vi "TargetControllers.vi"() -> ()   [LabVIEW 2024]
uses:
  <vilib>/platform/TimedLoop/XDataNode/XDataNode.xnode
  <vilib>/Platform/TimedLoop/XDataNode/nitl_modes.ctl
  <vilib>/Platform/TimedLoop/XDataNode/XDNodeRunTimeDep.lvlib
  <vilib>/Platform/TimedLoop/XDataNode/wakeup.ctl
  <vilib>/Platform/TimedLoop/XDataNode/timing_clust.ctl
  <vilib>/Analysis/Matrix/NI_Matrix.lvlib
  subVIs_target/GlobalVariables.vi
  <vilib>/addons/Maxon Motor/EPOS2 CANopen/EPOS2 Support Files/Typedefs/EPOS2 Control Word PVM.ctl
  <vilib>/addons/Maxon Motor/EPOS2 CANopen/EPOS2 Library.lvlib
  <vilib>/Analysis/Matrix/Numeric/Conversions/Array To Matrix - RA2.vi
  <vilib>/addons/control/pid/NI_PID_pid.lvlib
  <vilib>/addons/control/pid/pid.llb/PID Output Rate Limiter (DBL Array).vi
  <vilib>/addons/Maxon Motor/EPOS2 CANopen/CANopen/sbCANopenBaseClass.lvclass
panel:
  out "Convert microsecond to second array":dbl[](array[numeric])
  out "Previous Tensions":dbl[](array[numeric])
  in  "Use pull-only friction compensation in feedforward control":bool=TRUE
  in  "Use linear tension/current model in feedforward control":bool=TRUE
  out "Motor velocities in ascending motor order":dbl[](array[numeric]) format="%.2f"
  out "Reinitialize PID all motors flags":bool[](array[boolean])
  out "maskForAllActiveMotors":bool[](array[boolean])
  out "NumTotalActiveMotors":i32
  out "Robot Control Mode Target Local":T1(radio)
  out "kneeActiveMotorNumbers":i32[](array[numeric])
  out "pelvisActiveMotorNumbers":i32[](array[numeric])
  out "trunkActiveMotorNumbers":i32[](array[numeric])
  out "NumActiveKneeMotors":i32
  out "NumActivePelvisMotors":i32
  out "NumActiveTrunkMotors":i32
  out "Velocity 5":dbl[](array[numeric])
  out "Velocity 3":dbl[](array[numeric])
  out "Velocity 2":dbl[](array[numeric])
  out "Motor order":i32[](array[numeric])=[3, 6, 9, 12, 2, 7, 8, 13, 4, 5, 10, 11, 1, 14]
  out "maskForKneeMotors":bool[](array[boolean])
  out "maskForPelvisMotors":bool[](array[boolean])
  out "maskForTrunkMotors":bool[](array[boolean])
  out "Vicon Sync":dbl format="%0.2f"
  out "True_Knees":bool=TRUE
  out "final current":dbl[](array[numeric])
  out "Pelvis Forces Enabled":bool=TRUE
  out "canERROR":errorcluster[](array[cluster])
  in  "CANcurrent 2":dbl[](array[numeric])
  out "Low-Level Controller Finished Late?":bool
  out "CANcurrent":dbl[](array[numeric])
  out "Read Late":bool
  out "Read Time":i64
  out "I32":i32
  out "Write Late":bool
  out "Write Time":i64
  out "canID":refnum<class "sbCANopenBaseClass.lvclass">[](array[class])
  out "nMotorsCAN":i32
  out "AcT":dbl[](array[numeric])
  out "Period_HL":dbl format="%.2f"
  out "Current Tension":dbl[](array[numeric])
  in  "Stop":bool
  out "UseATI":bool
  out "PID loop duration [us]":i64
  # "Note before running this VI:\n1. Ensure correct motors are selected \nusing MotorsToUse.\n2. Connected load cells should have \nthe same order as MotorsToUse.\n\n-------- Do appropriate transformation in CONSTS LL and HL VIs -----------\n(especially MotorsPos_wrt_Markers )"
  # "Motor Order \n(Trunk, Pelvis, Pelvis_M, Leg)\n3\n6\n9\n12\n2\n7\n8\n13\n4\n5\n10\n11\n1\n14"
  # "This part reads\nmotors in order from\nTrunk, pel, etc, and not\nthe motor # order 1-14. \n\nAlso, the code motor number\nis 1 less than the labeled motor \nnumber (e.g., motor 1 is 0)."
types:
  T1 = enum32{"Idle", "Constant", "Live Forces", "Single Motor", "Constant Feedforward"}
  T2 = typedef "EPOS2 Library.lvlib/EPOS2 Control Word PVM.ctl" = cluster{"Switch On":bool, "Enable Voltage":bool, "Quick Stop":bool, "Enable Operation":bool, "Reserved 0":bool, "Reserved 1":bool, "Reserved 2":bool, "Fault Reset":bool, "Halt":bool}
  T3 = typedef "XDNodeRunTimeDep.lvlib/timing_clust.ctl" = cluster{"Expected End [f-1]":u64, "Actual End [f-1]":u64, "Finished Late? [f-1]":bool, "Expected End [i-1]":u64, "Actual End [i-1]":u64, "Finished Late? [i-1]":bool, "Expected Start [i]":u64, "Actual Start [i]":u64, "Expected Start [f]":u64, "Actual Start [f]":u64, "Source Name":string, "Structure Name":string, "Period":i64, "Deadline":i64, "Offset":i64, "Start":i64, "Priority":i32, "Timeout":i32, "Mode":T4, "Wakeup Reason":T5, "Error":errorcluster, "Source Type":string, "Secondary Source Type":string, "Global End Time":u64, "Global Start Time":u64, "Frame Duration":u64, "Iteration Duration":u64, "Assigned CPU":i32, "I/O Scan Engine Mode":u32}
  T4 = typedef "XDNodeRunTimeDep.lvlib/nitl_modes.ctl" = enum32{"No Change", "Process missed periods, maintain original phase", "Discard missed periods, maintain original phase", "Process missed periods, ignore original phase", "Discard missed periods, ignore original phase"}
  T5 = typedef "XDNodeRunTimeDep.lvlib/wakeup.ctl" = enum32{"Normal", "Aborted", "Asynchronous wakeup", "Timing source error", "Timed loop error", "Timeout"}
  T6 = typedef "constants_LL.ctl" = cluster{"zero array":dbl[], "decRate_ff":dbl[], "Motor constants":dbl[], "PID gains":cluster{"proportional gain (Kc)":dbl, "integral time (Ti, min)":dbl, "derivative time (Td, min)":dbl}[], "decRate _fb":dbl[], "PID_OP_upLim":dbl, "nMotors":i32, "PID_betas":dbl[], "filtOrder":i32, "filtLowCutFreq":dbl, "filtSamplFreq":dbl, "whichMotors":i32[], "nMotors 1":i32, "nMotors 2":i32, "Motor constants pel":dbl[], "Motor constants trunk":dbl[], "whichMotors 1":i32[], "whichMotors 2":i32[], "zero array pel":dbl[], "decRate_ff pel":dbl[], "decRate _fb pel":dbl[], "PID_betas pel":dbl[], "whichMotors 3":i32[], "nMotors 3":i32, "Motor constants knees":dbl[], "zero array knees":dbl[], "decRate_ff knees":dbl[], "decRate _fb knees":dbl[], "PID_betas knees":dbl[]}
  T7 = typedef "NI_Matrix.lvlib/RealMatrix.ctl" = dbl[][]
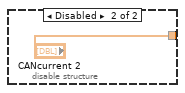
[diagram p2: hidden frame]
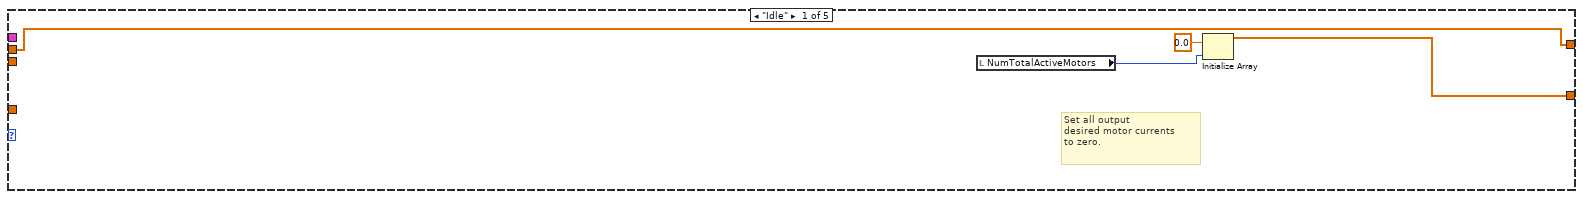
[diagram p4: hidden frame]
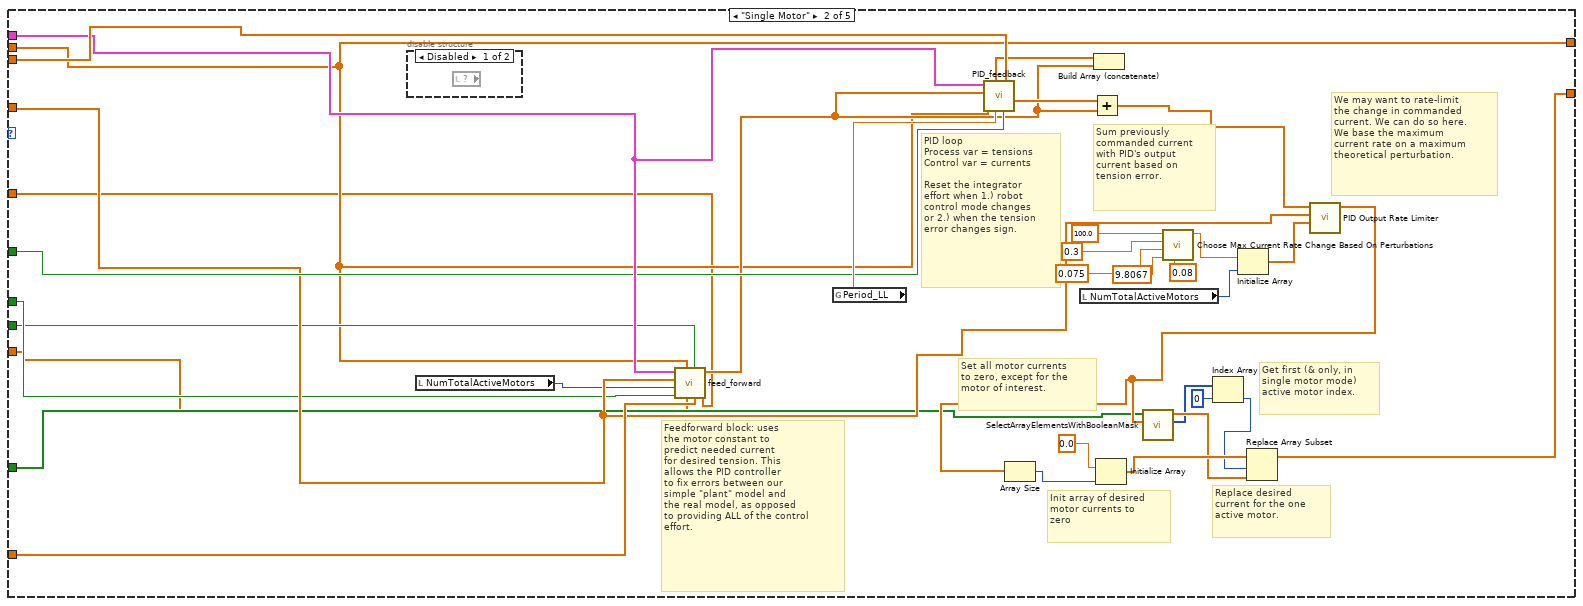
[diagram p5: hidden frame]
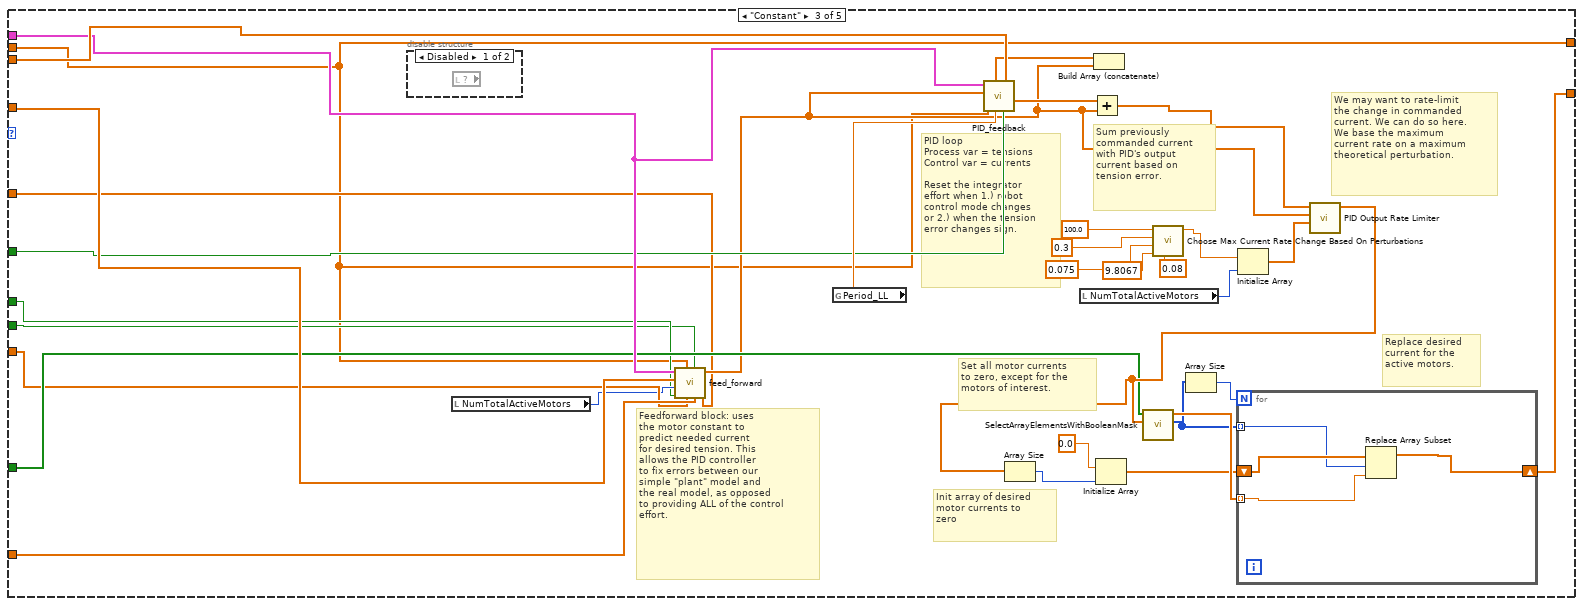
[diagram p7: hidden frame]
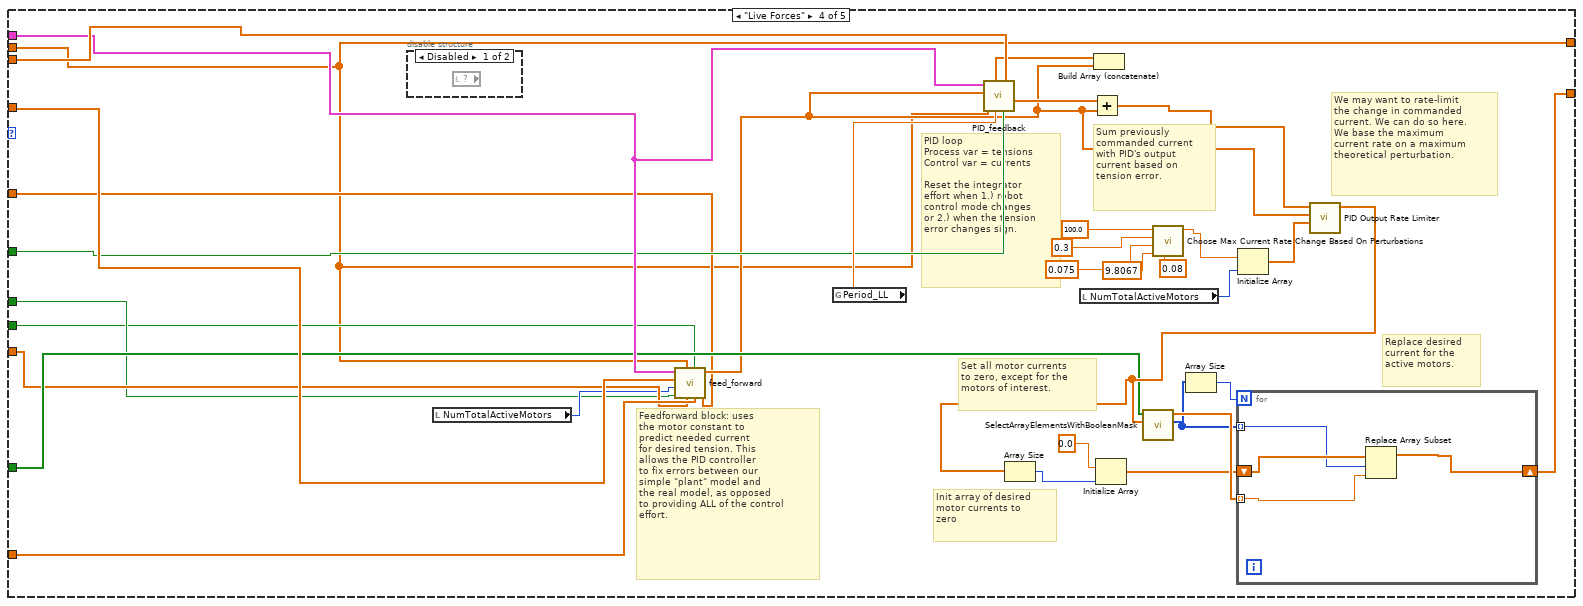
[diagram p9: hidden frame]
diagram:
  n1 = flat-sequence {
    tunnel: [w64] -> w17
    tunnel: [w62] -> w16
    tunnel: [w58] -> w15
    tunnel: [w56] -> w14
    tunnel: [w55] -> w13
    tunnel: [w49] -> w10
    tunnel: [w48] -> w9
    tunnel: w17 -> [w113]
    tunnel: w16 -> [_]
    tunnel: w15 -> [_]
    tunnel: w14 -> [w87]
    tunnel: w13 -> [w86]
    tunnel: [w87] -> w12
    tunnel: [w86] -> w11
    tunnel: w10 -> [w85]
    tunnel: w9 -> [w96]
    tunnel: [w97] -> w8
    tunnel: [w85] -> w7
    tunnel: [w96] -> w6
    tunnel: [w92] -> w2
    tunnel: [w91] -> w1
    tunnel: w12 -> [w383]
    tunnel: w11 -> [w382]
    tunnel: w8 -> [w379]
    tunnel: w7 -> [w378]
    tunnel: w6 -> [w377]
    tunnel: [w379] -> w5
    tunnel: [w376] -> w4
    tunnel: [w375] -> w3
    tunnel: w2 -> [w374]
    tunnel: w1 -> [w373]
    tunnel: w5 -> [w394]
    tunnel: w4 -> [w393]
    tunnel: w3 -> [w392]
    frame #0 {
      w44 = TRUE
      w46 = TRUE
      w57 = refnum<k21> "LEDTrust"  # DAQmx Task Name
      w63 = dbl[][] [[-1.3915001098602042, -96.36354731251453, 1.4901268489488144, 95.80055650167623, 0.11513435812043361, -0.20957134618573833], [-0.15155726034970227, -54.43374806490713, -0.3124157679711426, -56.28095342773552, -2.859114029977124, 103.37942505940691], [135.67639082873404, -1.227548634927782, 136.40217860533392, -2.4579984396752574, 136.3751481938431, -5.182267660606754], [-2.217796179322478, -0.3587679442089546, 2.274983310429265, -0.42200713926637096, -0.04878150351528989, 0.7012551466653533], [-1.289313295754956, 0.6617253849307168, -1.3327588652039173, -0.632747230304039, 2.4993576210336226, -0.09390740213198005], [-0.003620332273444647, -1.4342719694352277, -0.021014064916045613, -1.406174049990865, 0.009761043049281059, -1.3430405096008415]]  # Callibration Matrix Sensor ID: FT5769
      w61 = FALSE ("ATIConnected")
      # "This is the startup frame. \nAll code in this frame runs once \nat startup."
      # "At startup, we reinitialize\nthe PID controller to zero\nout the integrator."
      # "The current CAN Initialize assumes \na fixed order of motors, e.g. the first 4 are\n for the trunk, the next 8 are for the \npelvis, and the last two are for the knees. \nI added an int[] output that reports the order\nof the motor numbers."
      # "The low-level (LL) constants include \nmotor constants, PID constants for the tension loop\n, other?"
      # "CAN_motorselect.vi selects only\nthe motors we need given the flags \nof UsingTrunk, UsingPelvisPlanar, \nUsingPelvisMoments, and UsingKnees.\nOne idea: turn them all on and only \nwrite non-zero currents to those we need."
      # "Can_Initialize3.vi appears to\ninitialize all 14 motors"
      # "Low Level Constants: \nPID parameters\nMotor constants"
      # "LED Trust"
      # "Operation Mode\nEnabled"
      # "Legs"
      # "Pelvis-Forces/Moments"
      # "Pelvis-Planar"
      # "Trunk"
      # "Operation Mode\nDisabled"
      # "Initialize/\nPreOperation"
      n2 = call "CAN_initialize3.vi"() -> ("Array 2"=w41:errorcluster[], "Array"=w43:refnum<class "sbCANopenBaseClass.lvclass">[], "Motor order"=→"Motor order":i32[])  [unwired: 3 in]
      n3 = shared-variable "NI-PXIe8880-2F170198\\variables_AlwaysInUse - networkPublished.lvlib\\Use Vicon"(w61) -> ()  [unwired: 1 in, 1 out]
      n4 = shared-variable "NI-PXIe8880-2F170198\\variables_ToSetPID - networkPublished.lvlib\\SetPID"(w61) -> ()  [unwired: 1 in, 1 out]
      n5 = shared-variable "NI-PXIe8880-2F170198\\variables_AlwaysInUse - networkPublished.lvlib\\Use ATI"(w61) -> ()  [unwired: 1 in, 1 out]
      n6 = call "CAN_MotorSelect.vi"("Trunk"=TRUE, "Nodes In"=w43, "Pelvis"=w46, "Pelvis_Moments"=TRUE, "Legs"=w44, "Error In"=w41) -> ("maskForTrunkMotors"=w25:bool[], "Nodes Out"=w42:refnum<class "sbCANopenBaseClass.lvclass">[], "nMotorsCAN"=w39:i32, "maskForKneeMotors"=w23:bool[], "CANmotorsuse"=w38:bool[], "Error Out"=w40:errorcluster[], "maskForPelvisMotors"=w24:bool[])  [unwired: 3 in]
      "nMotorsCAN" <- w39
      "maskForTrunkMotors" <- w25
      "maskForPelvisMotors" <- w24
      "maskForKneeMotors" <- w23
      n7 = local read "Motor order"() -> (w33:i32[])
      n8 = for {
        N: w39 -> [_]
        tunnel: [w79] -> w53 mode=indexing
        tunnel: w42 -> [w78] mode=indexing
        tunnel: w40 -> [w77] mode=indexing
        tunnel: [w75] -> w54 mode=indexing
        n9 = Wait (ms)(milliseconds to wait=u32 100) -> ()  [unwired: 1 out]
        n10 = call "CAN_enableOFF.vi"("error in (no error)"=w77, "Current"=0, "sbCANopenBaseClass in"=w78) -> ("error out"=w79:errorcluster, "CANopen Session Out"=w75:refnum<class "sbCANopenBaseClass.lvclass">)  [unwired: 1 in]
      }
      n11 = local write "Stop"(FALSE ("Stop")) -> ()
      n12 = call "SelectArrayElementsWithBooleanMask.vi"("InputArray"=w33, "BooleanMaskArray"=w24) -> ("OutputArray"=→"pelvisActiveMotorNumbers":dbl[])  [unwired: 8 in, 1 out]
      n13 = call "SelectArrayElementsWithBooleanMask.vi"("InputArray"=w33, "BooleanMaskArray"=w25) -> ("OutputArray"=→"trunkActiveMotorNumbers":dbl[])  [unwired: 8 in, 1 out]
      n14 = call "SelectArrayElementsWithBooleanMask.vi"("InputArray"=w33, "BooleanMaskArray"=w23) -> ("OutputArray"=→"kneeActiveMotorNumbers":dbl[])  [unwired: 8 in, 1 out]
      n15 = shared-variable "NI-PXIe8880-2F170198\\variables_AlwaysInUse - networkPublished.lvlib\\directTension"(0.0 ("directTension")) -> ()  [unwired: 1 in, 1 out]
      n16 = call "Sum_True_Elements_In_Boolean_Array.vi"("InputBooleanArray"=w23) -> ("NumTruesInArray"=w27:i32)  [unwired: 10 in]
      "NumActiveKneeMotors" <- w27
      n17 = call "Sum_True_Elements_In_Boolean_Array.vi"("InputBooleanArray"=w25) -> ("NumTruesInArray"=w29:i32)  [unwired: 10 in]
      "NumActiveTrunkMotors" <- w29
      n18 = call "Sum_True_Elements_In_Boolean_Array.vi"("InputBooleanArray"=w24) -> ("NumTruesInArray"=w28:i32)  [unwired: 10 in]
      "NumActivePelvisMotors" <- w28
      n19 = Bundle By Name(cluster=T2 {"Switch On"=TRUE, "Enable Voltage"=TRUE, "Quick Stop"=TRUE, "Enable Operation"=TRUE, "Reserved 0"=FALSE, "Reserved 1"=FALSE, "Reserved 2"=FALSE, "Fault Reset"=FALSE, "Halt"=FALSE} ("Control Word"), "Switch On"=TRUE) -> (w50:T2)
      n20 = Add(x=w29, y=w28) -> (x+y=w26:i32)
      n21 = for {
        N: w39 -> [_]
        tunnel: w54 -> [w70]
        tunnel: w53 -> [w69]
        tunnel: w50 -> [w65]
        tunnel: [w67] -> w49 mode=indexing
        tunnel: [w66] -> w48 mode=indexing
        i -> [w71]
        # "Writes current = 0 to all motors.\nTURNING ON the first 4 boolean values \nin the \"otuput cluster\" variable of CAN_MotorControl2.vi\nputs the CAN node in the correct mode for reading\nPDOs (current, velocity, position, etc.)"
        n22 = Wait (ms)(milliseconds to wait=u32 100) -> ()  [unwired: 1 out]
        n23 = Index Array(array=w70, index=w71) -> (element=w74:refnum<class "sbCANopenBaseClass.lvclass">)
        n24 = Index Array(array=w69, index=w71) -> (element=w68:errorcluster)
        n25 = call "CAN_MotorControl2.vi"("output cluster"=w65, "sbCANopenBaseClass in"=w74, "Current"=0, "error in (no error)"=w68) -> ("CANopen Session Out"=w67:refnum<class "sbCANopenBaseClass.lvclass">, "error out"=w66:errorcluster)  [unwired: 2 in]
      }
      n26 = Add(x=w26, y=w27) -> (x+y=w18:i32)
      "NumTotalActiveMotors" <- w18
      n27 = Or(x=w25, y=w24) -> (x .or. y?=w22:bool[])
      n28 = Or(x=w22, y=w23) -> (x .or. y?=→"maskForAllActiveMotors":bool[])
      n29 = local read "NumActiveKneeMotors"() -> (w34:i32)
      n30 = local read "NumActivePelvisMotors"() -> (w35:i32)
      n31 = local read "NumActiveTrunkMotors"() -> (w36:i32)
      n32 = Initialize Array(TRUE, w18) -> (→"Reinitialize PID all motors flags":bool[])
      n33 = call "constants_LL.vi"("NumKneeMotorsInUse"=w34, "NumPelvisMotorsInUse"=w35, "MotorsInUse"=w38, "NumTrunkMotorsInUse"=w36) -> ("Constants LL"=w64:T6)  [unwired: 7 in]
      n34 = call-poly <vilib>:"Array To Matrix.vi"("Real 2D Array"=w63) -> ("Real Matrix"=w62:T7)
      n35 = call <vilib>:"DAQmx Start Task.vi"("task/channels in"=w57) -> ("task out"=w56:refnum<k21>, "error out"=w55:errorcluster)  [unwired: 13 in]
      n36 = Tick Count (ms)() -> (millisecond timer value=w58:u32)
      "Pelvis Forces Enabled" <- w46
      "True_Knees" <- w44
    }
    frame #1 {
      w93 = i64 5000  # @ 200Hz
      w110 = i64 2500  # @ 1000Hz
      # "Used to convert N/us to N/s"
      # "Period for reading \nCAN data (in us)"
      # "This is the primary frame of the code. \nAll timed loops are in this frame. \nFrom top to bottom:\n1.) Write CAN loop: sends desired motor currents to the motor controllers.\n2.) Read CAN loop: seems to only read motor velocity (RPM). Note that tension sensors \nare read in the LL controller loop. \n3.)  Low level controller loop: based on desired tensions, uses feedforward control \n(special motor constant * current = tension) and PID feedback control on tensions to set desired motor\ncurrents."
      # "All motor currents are \ninitialized at 0 A"
      # "Here is the output of CAN nodes \nwith all the motors. All of these motors\nare in Current mode and are enabled."
      # "Rob 3/7/23: Was 2000 us delay (500Hz), \nslowing to 2,500 us delay (400 Hz)"
      # "Rob 3/7/23: Was 5000 us delay, \nslowing to 10,000."
      # "Global Variables are made by saving a separate VI\nright-click and explore to see it"
      # "These are typedefs below.\nAdjustable in project list"
      # "d1: time, cT, dT\n\nd4: d1, fN, data, QP_error\n\ndata: dFM, cFM, dFMNF, ..."
      # "About 750Hz"
      # "CAN protocol does not like local variables for some reason. Use these long wires to connect"
      # "uses 0 to 13 for motors"
      # "sec"
      n37 = node-c288(i64 1000 ("Period")) -> (w95:T3)  [unwired: 3 in]
      n38 = timed-loop {
        timing: w95 -> [_]
        timing-out: [_] -> w94
        tunnel: w85 -> [w122]
        tunnel: w96 -> [w123]
        stop <- w130 stop-if-true
        # "The motor velocities are in the order of the NodeIDs. \nRe-order to ascending motor numbers."
        # "GearRatio"
        # "Read CAN"
        n39 = node-c288() -> (→"Read Late":bool, →"Read Time":i64)  [unwired: 1 in, 1 out]
        n40 = local read "NumTotalActiveMotors"() -> (w124:i32)
        n41 = for {
          N: w124 -> [_]
          tunnel: [w140] -> w126 mode=indexing
          tunnel: w122 -> [w139] mode=indexing
          tunnel: w123 -> [w138] mode=indexing
          n42 = call-dynamic "sdCANopenPDOread.vi"("error in (no error)"=w138, "PDO Number"=u8 1, "sbCANopenBaseClass in"=w139) -> ("Data"=w141:u8[])  [unwired: 6 in, 2 out]
          n43 = Split 1D Array(array=w141, index=4) -> (first subarray=w137:u8[])  [unwired: 1 out]
          n44 = call <vilib>:"sdCANutility4xU8toI32.vi"("Array 4 U8"=w137) -> ("I32"=w140:i32)
          "I32" <- w140
        }
        n45 = Initialize Array(14.0 ("element"), w124) -> (w127:dbl[])
        n46 = local read "NumTotalActiveMotors"() -> (w119:i32)
        n47 = local read "Motor order"() -> (w120:i32[])
        n48 = Divide(x=w126, y=w127) -> (x/y=w121:dbl[])
        n49 = Initialize Array(0.0 ("element"), w119) -> (w117:dbl[])
        n50 = for {
          tunnel: w121 -> [w132] mode=indexing
          tunnel: w120 -> [w136] mode=indexing
          shift-right: [w131] -> w116
          shift-left: w117 -> [w134]
          # "When storing in ascending motor\norder, the index is just the motor \nnumber - 1."
          n51 = Subtract(x=w136, y=1) -> (x-y=w133:i32)
          n52 = Replace Array Subset(array=w134, new element=w132, index=w133) -> (w131:dbl[])
        }
        "Motor velocities in ascending motor order" <- w116
        n53 = local read "Stop"() -> (w130:bool)
        n54 = node-c288() -> ()  [unwired: 1 in, 1 out]
      }
      n55 = node-c288() -> (w105:T3)  [unwired: 3 in]
      n56 = Bundle By Name(cluster=T2 {"Switch On"=TRUE, "Enable Voltage"=TRUE, "Quick Stop"=TRUE, "Enable Operation"=TRUE, "Reserved 0"=FALSE, "Reserved 1"=FALSE, "Reserved 2"=FALSE, "Fault Reset"=FALSE, "Halt"=FALSE} ("Control Word"), "Switch On"=TRUE) -> (w101:T2)
      n57 = timed-loop {
        tunnel: w96 -> [w159]
        tunnel: [w157] -> _
        timing: w105 -> [_]
        timing-out: [_] -> w104
        tunnel: w101 -> [w155]
        tunnel: w85 -> [w160]
        tunnel: [w156] -> _
        stop <- w154 stop-if-true
        # "Here, the latest computed motor currents are \nsent to each motor via the CAN communication protocol."
        # "Write CAN"
        n58 = node-c288() -> (→"Write Late":bool, →"Write Time":i64)  [unwired: 1 in, 2 out]
        n59 = disable-structure shown="Enabled" {
          disable-tunnel: [w162 "CANcurrent 2"] -> w152
          frame Enabled {
            n60 = local read "CANcurrent"() -> (w162:dbl[])
          }
          frame Disabled {
          }
        }
        n61 = local read "nMotorsCAN"() -> (w153:i32)
        n62 = for {
          N: w153 -> [_]
          tunnel: [w170] -> w156 mode=indexing
          tunnel: [w171] -> w157 mode=indexing
          tunnel: w160 -> [w172] mode=indexing
          tunnel: w159 -> [w173] mode=indexing
          tunnel: w155 -> [w169]
          tunnel: w152 -> [w168] mode=indexing
          n63 = call "CAN_MotorControl2.vi"("output cluster"=w169, "sbCANopenBaseClass in"=w172, "Current"=w168, "error in (no error)"=w173) -> ("CANopen Session Out"=w170:refnum<class "sbCANopenBaseClass.lvclass">, "error out"=w171:errorcluster)  [unwired: 2 in]
        }
        "canID" <- w156
        "canERROR" <- w157
        n64 = local read "Stop"() -> (w154:bool)
        n65 = node-c288() -> ()  [unwired: 1 in, 1 out]
      }
      n66 = local read "NumTotalActiveMotors"() -> (w83:i32)
      n67 = local read "NumTotalActiveMotors"() -> (w89:i32)
      n68 = Initialize Array(1000000.0 ("element"), w83) -> (→"Convert microsecond to second array":dbl[])
      n69 = call <vilib>:"DAQmx Start Task.vi"("task/channels in"=refnum<k21> "SCI_TenSen") -> ("task out"=w100:refnum<k21>, "error out"=w99:errorcluster)  [unwired: 13 in]
      n70 = Initialize Array(0.0 ("element"), w89) -> (w88:dbl[])
      n71 = node-c288(w110) -> (w115:T3)  [unwired: 3 in]
      n72 = timed-loop "Timed Loop" {
        timing: w115 -> [_]
        timing-out: [_] -> w114
        shift-right: [w194] -> _
        shift-left: w88 -> [w207]
        shift-right: [w203] -> _
        shift-left: w113 -> [w212]
        tunnel: w99 -> [w188]
        tunnel: [w206] -> w91
        shift-right: [w205] -> w92
        shift-left: w100 -> [w205]
        stop <- "Stop" stop-if-true
        # "Do a \"quick and dirty\" approximation of \nchange in desired tension, in units of \nN/second. We approximate the loop time \nwith the previous loop time."
        # "Desired tensions [N]"
        # "Only read velocities IF we're using the pull comp. \nOtherwise, output 0 velocities.\nPROBLEM: reading is VERY slow, so if we activate this, \nour control loop performance tanks. Need to switch to PDO reads, currently SDO."
        # "CANcurrent: the \nvalues sent to the\nmotors over CAN."
        # "Our CAN nodes are \nordered in a certain way, \nwhereas our desired currents\nare ordered in ascending\norder. We must reorder them to\nmatch the CAN node order."
        # "Set the current robot control mode state.\n\nAlso, determine whether or not the robot high-level \ncontroller has switched states. We will use this information\nas whenever we change states, we want to zero the \nPID integrator effort. If the state has changed, output\n\"true\" to indicate that we want to reset the integrator."
        # "The ActiveMotorsFlags is a boolean mask\nwith dimension 14x1. All motors with a \nfalse will have their desired currents set to\n0. Note that this flag is set in the HostMain\nVI on the PC and depends on the robot \ncontrol mode."
        # "This is a \"friction compensation\"\nTENSION that was never fully \nimplemented."
        # "Below: motor selection masks\nfor all of the different robot modes."
        # "Convert from the int version of \nthe robot control mode (a global variable)\nback to a radio button format for clarity."
        # "DesiredTensionsX, where X is Trunk, \nPelvis, or Knees is a double array \nwith the number of elements equal to \nthe number of needed motors for that \nsegment. The"
        # "Feedforward motor\nfriction compensation \nin V (set to 0)"
        # "Here, tension\nvector is ordered\nby strain gauge \nnumber: 1,2,3,4,...\nand is thus \nin ascending\norder."
        # "This case structure determines desired currents for ALL motors. All motors \nnot included in the relevant state's motor mask will receive desired currents \nof zero."
        # "The DAQ is running\nthe \"SCI_TenSen\" \n(tension sensing) \ntask, meaning it \nwill read the tension\nsensors. The task \nname is set above (trace the Refnum in\ninput to \nAnalog_IP_Data.vi)"
        # "fix this"
        # "Current tension is initially read here!"
        # "Please be aware that ATI not considered for UseATI=true"
        # "Low Level Tension Controller"
        n73 = node-c288() -> (→"PID loop duration [us]":i64, →"Low-Level Controller Finished Late?":bool)  [unwired: 1 in]
        n74 = shared-variable "NI-PXIe8880-2F170198\\variables_AlwaysInUse - networkPublished.lvlib\\Use ATI"() -> (→"UseATI":bool)  [unwired: 1 in, 1 out]
        n75 = shared-variable "NI-PXIe8880-2F170198\\variables_ToSetPID - networkPublished.lvlib\\SetPID"() -> (w211:bool)  [unwired: 1 in, 1 out]
        n76 = case shown="True" w211 {
          tunnel: w212 -> [w222 w225]
          tunnel: [w222 w224] -> w203
          frame False {
          }
          frame True {
            n77 = shared-variable "NI-PXIe8880-2F170198\\variables_ToSetPID - networkPublished.lvlib\\pidGains"() -> (w223:dbl[])  [unwired: 1 in, 1 out]
            n78 = call "SetPIDGains.vi"("pidGains"=w223, "Constants LL in"=w225) -> ("Constants LL out"=w224:T6)  [unwired: 9 in]
          }
        }
        n79 = local read "Robot Control Mode Target Local"() -> (w197:T1)
        n80 = shared-variable "NI-PXIe8880-2F170198\\variables_Unity_Data.lvlib\\RobotControlModeAsInt"() -> (w198:i32)  [unwired: 1 in, 1 out]
        "Robot Control Mode Target Local" <- w198
        n81 = Not Equal?(x=w198, y=w197) -> (x != y?=w196:bool)
        n82 = call "Analog_IP_Data.vi"("Refnum in"=w205, "error in (no error)"=w188, "Constants LL"=w203) -> ("Tension Sensors Data"=w195:dbl[], "error out"=w206:errorcluster, "Vicon Sync"=→"Vicon Sync":dbl)  [unwired: 1 in, 5 out]
        "Current Tension" <- w195
        "AcT" <- w195
        n83 = local read "Motor velocities in ascending motor order"() -> (w185:dbl[])
        n84 = shared-variable "NI-PXIe8880-2F170198\\variables_Unity_Data.lvlib\\DesiredTensionsInAscendingMotorOrder"() -> (w182:dbl[])  [unwired: 1 in, 1 out]
        n85 = local read "Previous Tensions"() -> (w181:dbl[])
        n86 = shared-variable "NI-PXIe8880-2F170198\\variables_Unity_Data.lvlib\\AllCurrentTensions"(w195) -> ()  [unwired: 1 in, 1 out]
        n87 = local read "Convert microsecond to second array"() -> (w177:dbl[])
        n88 = local read "PID loop duration [us]"() -> (w180:i64)
        n89 = Subtract(x=w182, y=w181) -> (x-y=w179:dbl[])
        n90 = local read "Robot Control Mode Target Local"() -> (w202:T1)
        n91 = local read "NumTotalActiveMotors"() -> (w201:i32)
        n92 = shared-variable "NI-PXIe8880-2F170198\\variables_Unity_Data.lvlib\\ActiveMotorsFlags"() -> (w199:bool[])  [unwired: 1 in, 1 out]
        n93 = Divide(x=w179, y=w180) -> (x/y=w178:dbl[])
        n94 = Multiply(x=w178, y=w177) -> (x*y=w176:dbl[])
        n95 = Initialize Array(40.0 ("element"), w201) -> (w200:dbl[])
        n96 = case shown="\"Constant Feedforward\"" w202 {
          tunnel: [w227 w262 w278 w314 w349] -> w194
          tunnel: w207 -> [_ w243 w294 w330 w360]
          tunnel: w195 -> [_ w261 w293 w329 _]
          tunnel: w203 -> [_ w259 w291 w327 w358]
          tunnel: w182 -> [w226 w231 w263 w299 w335]
          tunnel: w200 -> [_ w260 w292 w328 w359]
          tunnel: w199 -> [_ w242 w281 w317 w352]
          tunnel: w196 -> [_ w244 w282 w318 _]
          tunnel: w185 -> [_ w233 w268 w304 w339]
          tunnel: "Use linear tension/current model in feedforward control" -> [_ w234 w266 w302 _]
          tunnel: "Use pull-only friction compensation in feedforward control" -> [_ w232 w265 w301 _]
          tunnel: [w226 w231 w263 w299 w335] -> w183
          tunnel: w176 -> [_ w230 w264 w300 w336]
          frame "Idle" {
            # "Set all output \ndesired motor currents\nto zero."
            n97 = local read "NumTotalActiveMotors"() -> (w228:i32)
            n98 = Initialize Array(0.0 ("element"), w228) -> (w227:dbl[])
          }
          frame "Single Motor" {
            # "Replace desired\ncurrent for the one \nactive motor."
            # "Init array of desired \nmotor currents to \nzero"
            # "Get first (& only, in\nsingle motor mode)\nactive motor index."
            # "We may want to rate-limit\nthe change in commanded \ncurrent. We can do so here.\nWe base the maximum \ncurrent rate on a maximum\ntheoretical perturbation."
            # "Sum previously \ncommanded current\nwith PID's output \ncurrent based on \ntension error."
            # "PID loop\nProcess var = tensions\nControl var = currents\n\nReset the integrator\neffort when 1.) robot\ncontrol mode changes \nor 2.) when the tension\nerror changes sign."
            # "Feedforward block: uses\nthe motor constant to \npredict needed current \nfor desired tension. This\nallows the PID controller\nto fix errors between our \nsimple \"plant\" model and \nthe real model, as opposed\nto providing ALL of the control\neffort."
            # "Set all motor currents\nto zero, except for the \nmotor of interest."
            n99 = disable-structure shown="Disabled" {
              frame Disabled {
                n100 = local read item#-1() -> ()  [unwired: 1 out]
              }
              frame Enabled {
              }
            }
            n101 = local read "NumTotalActiveMotors"() -> (w235:i32)
            n102 = call "feed_forward.vi"("Desired tension velocities [N/s]"=w230, "frictionCompensationTensions"=w260, "Use pull-only friction compensation in feedforward"=w232, "Motor velocities (rpm)"=w233, "DesiredTensionsInAscendingMotorOrder"=w231, "Use linear tension/current modle in feedforward"=w234, "Num Total Active Motors"=w235, "lastCommandedMotorCurrent"=w243, "Constants LL"=w259) -> ("feedforwardPredictedMotorCurrents"=w241:dbl[])  [unwired: 2 in]
            n103 = global read "GlobalVariables.vi" "Period_LL"() -> (w257:dbl)
            n104 = call "PID_feedback.vi"("Reset PID and integrator Flag"=w244, "currentTensions"=w261, "dt (s)"=w257, "desiredTensions"=w231, "feedforwardCurrentsIn"=w241, "Constants LL"=w259) -> ("pidCurrentsOut"=w258:dbl[])  [unwired: 5 in]
            n105 = local read "NumTotalActiveMotors"() -> (w247:i32)
            n106 = Add(x=w258, y=w241) -> (x+y=w249:dbl[])
            n107 = Build Array (concatenate)(w258, w241) -> ()  [unwired: 1 out]
            n108 = call "Choose Max Current Rate Change Based On Perturbations.vi"("TypicalCurrentToTensionMotorConstant"=0.08, "GravityAccelConstant"=9.8067, "MinRampTimeForTrapezoidalPertInSeconds"=0.075, "MaxFractionOfBodyWeightPert"=0.3, "MaxSubjectMassForPertInKg"=100.0) -> ("maxCurrentSlopeRisingPhaseAmpsPerMinute"=w248:dbl)  [unwired: 6 in]
            n109 = Initialize Array(w248, w247) -> (w246:dbl[])
            n110 = call-poly <vilib>:"PID Output Rate Limiter.vi"("output rate (EGU/min)"=w246, "initial output"=w243, "input (controller output)"=w249) -> ("output"=w245:dbl[])  [unwired: 5 in, 1 out]
            n111 = Array Size(array=w245) -> (size(s)=w256:i32)
            n112 = Initialize Array(0.0 ("element"), w256) -> (w254:dbl[])
            n113 = call "SelectArrayElementsWithBooleanMask.vi"("InputArray"=w245, "BooleanMaskArray"=w242) -> ("trueIndices"=w252:i32[], "OutputArray"=w253:dbl[])  [unwired: 8 in]
            n114 = Index Array(array=w252, index=0) -> (element=w250:i32)
            n115 = Replace Array Subset(array=w254, new element=w253, index=w250) -> (w262:dbl[])
          }
          frame "Constant" {
            # "Replace desired\ncurrent for the \nactive motors."
            # "Init array of desired \nmotor currents to \nzero"
            # "We may want to rate-limit\nthe change in commanded \ncurrent. We can do so here.\nWe base the maximum \ncurrent rate on a maximum\ntheoretical perturbation."
            # "Sum previously \ncommanded current\nwith PID's output \ncurrent based on \ntension error."
            # "PID loop\nProcess var = tensions\nControl var = currents\n\nReset the integrator\neffort when 1.) robot\ncontrol mode changes \nor 2.) when the tension\nerror changes sign."
            # "Feedforward block: uses\nthe motor constant to \npredict needed current \nfor desired tension. This\nallows the PID controller\nto fix errors between our \nsimple \"plant\" model and \nthe real model, as opposed\nto providing ALL of the control\neffort."
            # "Set all motor currents\nto zero, except for the \nmotors of interest."
            n116 = disable-structure shown="Disabled" {
              frame Disabled {
                n117 = local read item#-1() -> ()  [unwired: 1 out]
              }
              frame Enabled {
              }
            }
            n118 = local read "NumTotalActiveMotors"() -> (w267:i32)
            n119 = call "feed_forward.vi"("Desired tension velocities [N/s]"=w264, "frictionCompensationTensions"=w292, "Use pull-only friction compensation in feedforward"=w265, "Motor velocities (rpm)"=w268, "DesiredTensionsInAscendingMotorOrder"=w263, "Use linear tension/current modle in feedforward"=w266, "Num Total Active Motors"=w267, "lastCommandedMotorCurrent"=w294, "Constants LL"=w291) -> ("feedforwardPredictedMotorCurrents"=w275:dbl[])  [unwired: 2 in]
            n120 = global read "GlobalVariables.vi" "Period_LL"() -> (w289:dbl)
            n121 = call "PID_feedback.vi"("Reset PID and integrator Flag"=w282, "currentTensions"=w293, "dt (s)"=w289, "desiredTensions"=w263, "feedforwardCurrentsIn"=w275, "Constants LL"=w291) -> ("pidCurrentsOut"=w290:dbl[])  [unwired: 5 in]
            n122 = local read "NumTotalActiveMotors"() -> (w285:i32)
            n123 = Add(x=w290, y=w275) -> (x+y=w286:dbl[])
            n124 = Build Array (concatenate)(w290, w275) -> ()  [unwired: 1 out]
            n125 = call "Choose Max Current Rate Change Based On Perturbations.vi"("TypicalCurrentToTensionMotorConstant"=0.08, "GravityAccelConstant"=9.8067, "MinRampTimeForTrapezoidalPertInSeconds"=0.075, "MaxFractionOfBodyWeightPert"=0.3, "MaxSubjectMassForPertInKg"=100.0) -> ("maxCurrentSlopeRisingPhaseAmpsPerMinute"=w269:dbl)  [unwired: 6 in]
            n126 = Initialize Array(w269, w285) -> (w284:dbl[])
            n127 = call-poly <vilib>:"PID Output Rate Limiter.vi"("output rate (EGU/min)"=w284, "initial output"=w275, "input (controller output)"=w286) -> ("output"=w283:dbl[])  [unwired: 5 in, 1 out]
            n128 = Array Size(array=w283) -> (size(s)=w280:i32)
            n129 = Initialize Array(0.0 ("element"), w280) -> (w279:dbl[])
            n130 = call "SelectArrayElementsWithBooleanMask.vi"("InputArray"=w283, "BooleanMaskArray"=w281) -> ("trueIndices"=w277:i32[], "OutputArray"=w287:dbl[])  [unwired: 8 in]
            n131 = Array Size(array=w277) -> (size(s)=w276:i32)
            n132 = for {
              N: w276 -> [_]
              tunnel: w277 -> [w296] mode=indexing
              shift-right: [w297] -> w278
              shift-left: w279 -> [w298]
              tunnel: w287 -> [w295] mode=indexing
              n133 = Replace Array Subset(array=w298, new element=w295, index=w296) -> (w297:dbl[])
            }
          }
          frame "Live Forces" {
            # "Replace desired\ncurrent for the \nactive motors."
            # "Init array of desired \nmotor currents to \nzero"
            # "We may want to rate-limit\nthe change in commanded \ncurrent. We can do so here.\nWe base the maximum \ncurrent rate on a maximum\ntheoretical perturbation."
            # "Sum previously \ncommanded current\nwith PID's output \ncurrent based on \ntension error."
            # "PID loop\nProcess var = tensions\nControl var = currents\n\nReset the integrator\neffort when 1.) robot\ncontrol mode changes \nor 2.) when the tension\nerror changes sign."
            # "Feedforward block: uses\nthe motor constant to \npredict needed current \nfor desired tension. This\nallows the PID controller\nto fix errors between our \nsimple \"plant\" model and \nthe real model, as opposed\nto providing ALL of the control\neffort."
            # "Set all motor currents\nto zero, except for the \nmotors of interest."
            n134 = disable-structure shown="Disabled" {
              frame Disabled {
                n135 = local read item#-1() -> ()  [unwired: 1 out]
              }
              frame Enabled {
              }
            }
            n136 = local read "NumTotalActiveMotors"() -> (w303:i32)
            n137 = call "feed_forward.vi"("Desired tension velocities [N/s]"=w300, "frictionCompensationTensions"=w328, "Use pull-only friction compensation in feedforward"=w301, "Motor velocities (rpm)"=w304, "DesiredTensionsInAscendingMotorOrder"=w299, "Use linear tension/current modle in feedforward"=w302, "Num Total Active Motors"=w303, "lastCommandedMotorCurrent"=w330, "Constants LL"=w327) -> ("feedforwardPredictedMotorCurrents"=w311:dbl[])  [unwired: 2 in]
            n138 = global read "GlobalVariables.vi" "Period_LL"() -> (w325:dbl)
            n139 = call "PID_feedback.vi"("Reset PID and integrator Flag"=w318, "currentTensions"=w329, "dt (s)"=w325, "desiredTensions"=w299, "feedforwardCurrentsIn"=w311, "Constants LL"=w327) -> ("pidCurrentsOut"=w326:dbl[])  [unwired: 5 in]
            n140 = local read "NumTotalActiveMotors"() -> (w321:i32)
            n141 = Add(x=w326, y=w311) -> (x+y=w322:dbl[])
            n142 = Build Array (concatenate)(w326, w311) -> ()  [unwired: 1 out]
            n143 = call "Choose Max Current Rate Change Based On Perturbations.vi"("TypicalCurrentToTensionMotorConstant"=0.08, "GravityAccelConstant"=9.8067, "MinRampTimeForTrapezoidalPertInSeconds"=0.075, "MaxFractionOfBodyWeightPert"=0.3, "MaxSubjectMassForPertInKg"=100.0) -> ("maxCurrentSlopeRisingPhaseAmpsPerMinute"=w305:dbl)  [unwired: 6 in]
            n144 = Initialize Array(w305, w321) -> (w320:dbl[])
            n145 = call-poly <vilib>:"PID Output Rate Limiter.vi"("output rate (EGU/min)"=w320, "initial output"=w311, "input (controller output)"=w322) -> ("output"=w319:dbl[])  [unwired: 5 in, 1 out]
            n146 = Array Size(array=w319) -> (size(s)=w316:i32)
            n147 = Initialize Array(0.0 ("element"), w316) -> (w315:dbl[])
            n148 = call "SelectArrayElementsWithBooleanMask.vi"("InputArray"=w319, "BooleanMaskArray"=w317) -> ("trueIndices"=w313:i32[], "OutputArray"=w323:dbl[])  [unwired: 8 in]
            n149 = Array Size(array=w313) -> (size(s)=w312:i32)
            n150 = for {
              N: w312 -> [_]
              tunnel: w313 -> [w332] mode=indexing
              shift-right: [w333] -> w314
              shift-left: w315 -> [w334]
              tunnel: w323 -> [w331] mode=indexing
              n151 = Replace Array Subset(array=w334, new element=w331, index=w332) -> (w333:dbl[])
            }
          }
          frame "Constant Feedforward" {
            # "Replace desired\ncurrent for the \nactive motors."
            # "Init array of desired \nmotor currents to \nzero"
            # "We may want to rate-limit\nthe change in commanded \ncurrent. We can do so here.\nWe base the maximum \ncurrent rate on a maximum\ntheoretical perturbation."
            # "Feedforward block: uses\nthe motor constant to \npredict needed current \nfor desired tension. This\nallows the PID controller\nto fix errors between our \nsimple \"plant\" model and \nthe real model, as opposed\nto providing ALL of the control\neffort."
            # "Set all motor currents\nto zero, except for the \nmotors of interest."
            n152 = disable-structure shown="Disabled" {
              frame Disabled {
                n153 = local read item#-1() -> ()  [unwired: 1 out]
              }
              frame Enabled {
              }
            }
            n154 = local read "NumTotalActiveMotors"() -> (w337:i32)
            n155 = call "feed_forward.vi"("Desired tension velocities [N/s]"=w336, "frictionCompensationTensions"=w359, "Motor velocities (rpm)"=w339, "DesiredTensionsInAscendingMotorOrder"=w335, "Use linear tension/current modle in feedforward"=TRUE, "Num Total Active Motors"=w337, "lastCommandedMotorCurrent"=w360, "Constants LL"=w358) -> ("feedforwardPredictedMotorCurrents"=w346:dbl[])  [unwired: 3 in]
            n156 = local read "NumTotalActiveMotors"() -> (w355:i32)
            n157 = call "Choose Max Current Rate Change Based On Perturbations.vi"("TypicalCurrentToTensionMotorConstant"=0.08, "GravityAccelConstant"=9.8067, "MinRampTimeForTrapezoidalPertInSeconds"=0.075, "MaxFractionOfBodyWeightPert"=0.3, "MaxSubjectMassForPertInKg"=100.0) -> ("maxCurrentSlopeRisingPhaseAmpsPerMinute"=w340:dbl)  [unwired: 6 in]
            n158 = Initialize Array(w340, w355) -> (w354:dbl[])
            n159 = call-poly <vilib>:"PID Output Rate Limiter.vi"("output rate (EGU/min)"=w354, "initial output"=w335, "input (controller output)"=w346) -> ("output"=w353:dbl[])  [unwired: 5 in, 1 out]
            n160 = Array Size(array=w353) -> (size(s)=w351:i32)
            n161 = Initialize Array(0.0 ("element"), w351) -> (w350:dbl[])
            n162 = call "SelectArrayElementsWithBooleanMask.vi"("InputArray"=w353, "BooleanMaskArray"=w352) -> ("trueIndices"=w348:i32[], "OutputArray"=w356:dbl[])  [unwired: 8 in]
            n163 = Array Size(array=w348) -> (size(s)=w347:i32)
            n164 = for {
              N: w347 -> [_]
              tunnel: w348 -> [w362] mode=indexing
              shift-right: [w363] -> w349
              shift-left: w350 -> [w364]
              tunnel: w356 -> [w361] mode=indexing
              n165 = Replace Array Subset(array=w364, new element=w361, index=w362) -> (w363:dbl[])
            }
          }
        }
        "final current" <- w194
        "Previous Tensions" <- w183
        n166 = local read "NumTotalActiveMotors"() -> (w193:i32)
        n167 = local read "Motor order"() -> (w190:i32[])
        n168 = Initialize Array(0.0 ("element"), w193) -> (w191:dbl[])
        n169 = call "ExpandArray.vi"("Array In"=w194) -> ()  [unwired: 10 in, 1 out]
        n170 = for {
          tunnel: w190 -> [w221] mode=indexing
          shift-right: [w215] -> w189
          shift-left: w191 -> [w216]
          shift-right: [w214] -> _
          shift-left: w194 -> [w214]
          i -> [w218]
          # "Replace CAN-node-ordered\ncurrent with the correct current."
          # "Get current corresponding\nwith motor number"
          # "Motor number is 1 greater\nthan its ascending index"
          n171 = Subtract(x=w221, y=1) -> (x-y=w219:i32)
          n172 = Index Array(array=w214, index=w219) -> (element=w217:dbl)
          n173 = Replace Array Subset(array=w216, new element=w217, index=w218) -> (w215:dbl[])
        }
        "CANcurrent" <- w189
        n174 = node-c288() -> ()  [unwired: 1 in, 1 out]
      }
      n175 = To Double Precision Float(number=w93) -> (double precision float=w109:dbl)
      n176 = To Double Precision Float(number=w110) -> (double precision float=w111:dbl)
      n177 = Divide(x=w111, y=1000000.0) -> (x/y=w106:dbl)
      n178 = global write "GlobalVariables.vi" "Period_LL"(w106) -> ()
      n179 = Divide(x=w109, y=1000000.0) -> (x/y=→"Period_HL":dbl)
      n180 = node-c288(w104) -> ()  [unwired: 1 out]
      n181 = node-c288(w94) -> ()  [unwired: 1 out]
      n182 = node-c288(w114) -> ()  [unwired: 1 out]
      n183 = local read "nMotorsCAN"() -> (w97:i32)
    }
    frame #2 {
      n184 = for {
        N: w379 -> [_]
        tunnel: [w391] -> w376 mode=indexing
        tunnel: [w389] -> w375 mode=indexing
        tunnel: w378 -> [w388] mode=indexing
        tunnel: w377 -> [w387] mode=indexing
        n185 = Wait (ms)(milliseconds to wait=u32 100) -> ()  [unwired: 1 out]
        n186 = call "CAN_enableOFF.vi"("error in (no error)"=w387, "Current"=0, "sbCANopenBaseClass in"=w388) -> ("error out"=w389:errorcluster, "CANopen Session Out"=w391:refnum<class "sbCANopenBaseClass.lvclass">)  [unwired: 1 in]
      }
      n187 = call <vilib>:"DAQmx Stop Task.vi"("task/channels in"=w383, "error in"=w382) -> ("task out"=w385:refnum<k21>, "error out"=w384:errorcluster)  [unwired: 12 in]
      n188 = call <vilib>:"DAQmx Stop Task.vi"("task/channels in"=w374, "error in"=w373) -> ("task out"=w380:refnum<k21>, "error out"=w381:errorcluster)  [unwired: 12 in]
      n189 = call <vilib>:"DAQmx Clear Task.vi"("task in"=w385, "error in"=w384) -> ()  [unwired: 13 in, 1 out]
      n190 = call <vilib>:"DAQmx Clear Task.vi"("task in"=w380, "error in"=w381) -> ()  [unwired: 13 in, 1 out]
    }
    frame #3 {
      n191 = for {
        N: w394 -> [_]
        tunnel: w393 -> [w396] mode=indexing
        tunnel: w392 -> [w395] mode=indexing
        n192 = call "CAN_STOP.vi"("error in"=w395, "CANopen Session In"=w396) -> ()  [unwired: 3 in, 1 out]
      }
    }
  }
